vi "grid_overlay and calculate grid size.vi"(11 "Image In":T1) -> (3 "Image Out":T1)   [LabVIEW 2017]
doc: "SciScan 1.2 160622"
uses:
  <vilib>/vision/Image Controls.llb/IMAQ Image.ctl
  GFG/GFGnumericGet.vi
  GFG/GFG library.lvlib
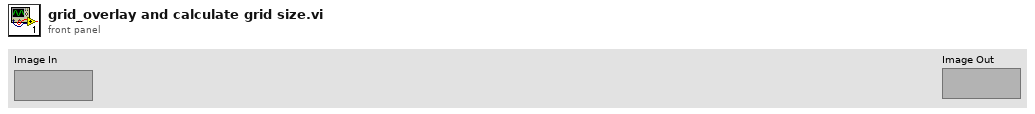
[diagram p1: front panel]
types:
  T1 = typedef "IMAQ Image.ctl" = refnum<image>
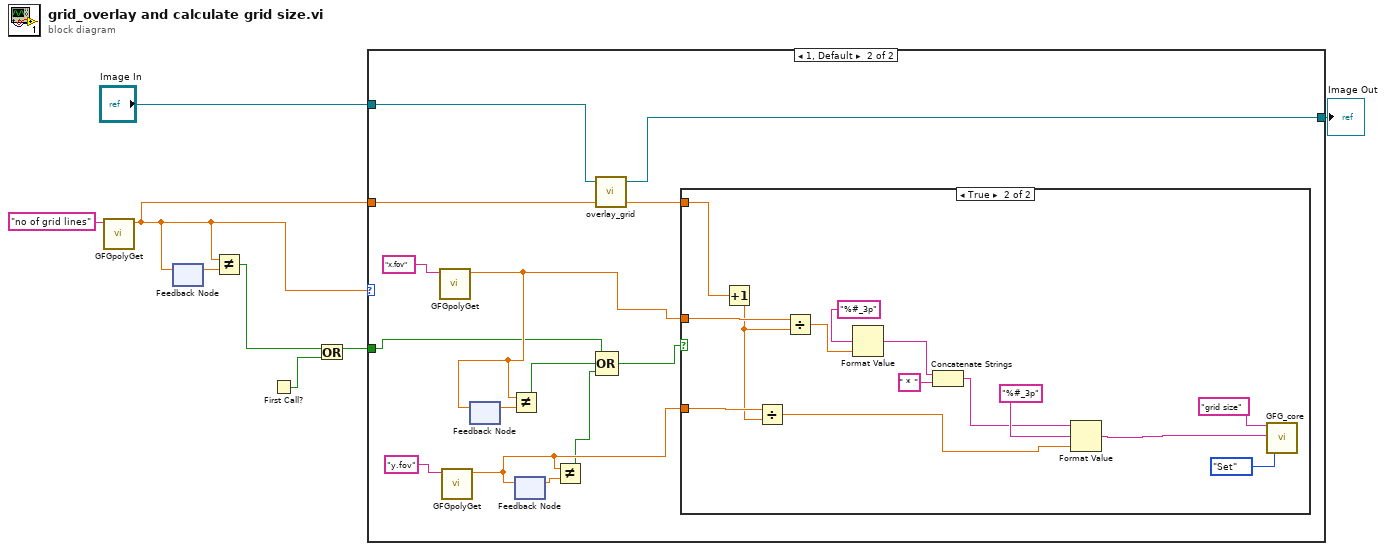
[diagram p0: block diagram]
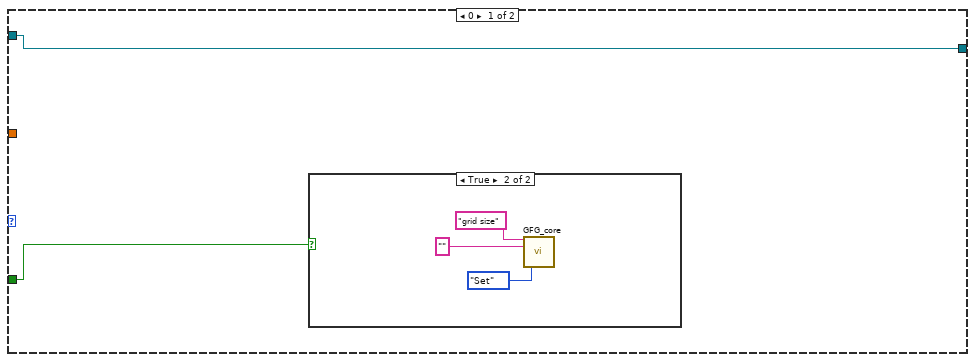
[diagram p2: hidden frame]
diagram:
  n1 = call-poly "GFGpolyGet.vi"("Variable Name in"="no of grid lines") -> ("Numeric"=w5:dbl)  [unwired: 8 in, 2 out]
  n2 = feedback-in #1(w5) -> ()
  n3 = feedback #1() -> (w4:dbl)  [unwired: 1 in]
  n4 = Not Equal?(x=w5, y=w4) -> (x != y?=w3:bool)
  n5 = First Call?() -> (First Call?: T/F=w1:bool)
  n6 = Or(x=w3, y=w1) -> (x .or. y?=w2:bool)
  n7 = case shown="1, Default" w5 {
    tunnel: "Image In" -> [w10 w26]
    tunnel: [w10 w25] -> w6
    tunnel: w5 -> [_ w24]
    tunnel: w2 -> [w9 w18]
    frame 0 {
      n8 = case shown="True" w9 {
        frame False {
        }
        frame True {
          n9 = call "GFG_core.vi"("Variable Name in"="grid size", "Variant in"="" ("f"), "Action"=enum16{"Init", "Set", "Get", "Clear"}."Set") -> ()  [unwired: 10 in, 7 out]
        }
      }
    }
    frame 1, Default {
      n10 = call-poly "GFGpolyGet.vi"("Variable Name in"="x.fov") -> ("Numeric"=w21:dbl)  [unwired: 8 in, 2 out]
      n11 = call-poly "GFGpolyGet.vi"("Variable Name in"="y.fov") -> ("Numeric"=w16:dbl)  [unwired: 8 in, 2 out]
      n12 = feedback #2() -> (w22:dbl)  [unwired: 1 in]
      n13 = feedback-in #2(w21) -> ()
      n14 = Not Equal?(x=w21, y=w22) -> (x != y?=w19:bool)
      n15 = feedback #3() -> (w17:dbl)  [unwired: 1 in]
      n16 = feedback-in #3(w16) -> ()
      n17 = Not Equal?(x=w16, y=w17) -> (x != y?=w15:bool)
      n18 = call "overlay_grid.vi"("no of grid lines"=w24, "Image In"=w26) -> ("Image Out"=w25:T1)  [unwired: 3 in]
      n19 = Compound Arithmetic op=OR(w18, w19, w15) -> (w14:bool)
      n20 = case shown="True" w14 {
        tunnel: w24 -> [_ w40]
        tunnel: w21 -> [_ w39]
        tunnel: w16 -> [_ w38]
        frame False {
        }
        frame True {
          n21 = Increment(x=w40) -> (x+1=w36:dbl)
          n22 = Divide(x=w38, y=w36) -> (x/y=w35:dbl)
          n23 = Divide(x=w39, y=w36) -> (x/y=w37:dbl)
          n24 = Format Value(format string="%#_3p", value (0)=w37) -> (output string=w33:string)  [unwired: 1 in]
          n25 = Concatenate Strings(w33, " * " ("string")) -> (w30:string)
          n26 = Format Value(string ("")=w30, format string="%#_3p", value (0)=w35) -> (output string=w27:string)
          n27 = call "GFG_core.vi"("Variable Name in"="grid size", "Variant in"=w27, "Action"=enum16{"Init", "Set", "Get", "Clear"}."Set") -> ()  [unwired: 10 in, 7 out]
        }
      }
    }
  }
  "Image Out" <- w6
